vi "TestExec.Run Executable and Rtn.vi"(7 "Vars":variant, 8 "error in":errorcluster, 9 "Timeout(s)":dbl=500.0 caption="Time Out(s)" format="%.2f", 10 "Log Dir":path=path "c:/MTE/Temp", 11 "Input":string[](array[string]) caption="Inputs") -> (0 "Error":errorcluster, 3 "RTN Data":T1 {"MeasData"."Status" items=["LOG", "PASS", "FAIL", "ERROR"]; "Attr"."Status" items=["LOG", "PASS", "FAIL", "ERROR"]; "Num"."Status" items=["LOG", "PASS", "FAIL", "ERROR"]})   [LabVIEW 2024]
uses:
  Cmd Exe/CmdExe.Output Error Check Setup.ctl
  Cmd Exe/CmdExe.Setup Params.ctl
  Results/Result.Measurement and Attribute Item Status.ctl
  Results/Result.Attribute.ctl
  Results/Result.Limit Type.ctl
  Results/Result.Numeric.ctl
  Results/Result XML/TestResult.SW Item.ctl
  Reports/Report.Result FileDataObject.ctl
  TestExec.Local Result Data.ctl
  Errors.lvlib
  <vilib>/KATE/Time/Time Utils.lvlib
  Results/Result.Measurement Item.ctl
  <vilib>/KATE/Files/File Utils.lvlib
panel:
  in  "Tab Control":enum32{"Execute", "Results"}(tab)
  out "Active":bool
  out "Sys Exec Commands":string
  out "Sys Exec STDOut":string
  out "Dur(s)":dbl caption="Duration(s)" format="%.3f"
  out "Rslt":u32(colorbox)=13816530 caption="Exe"
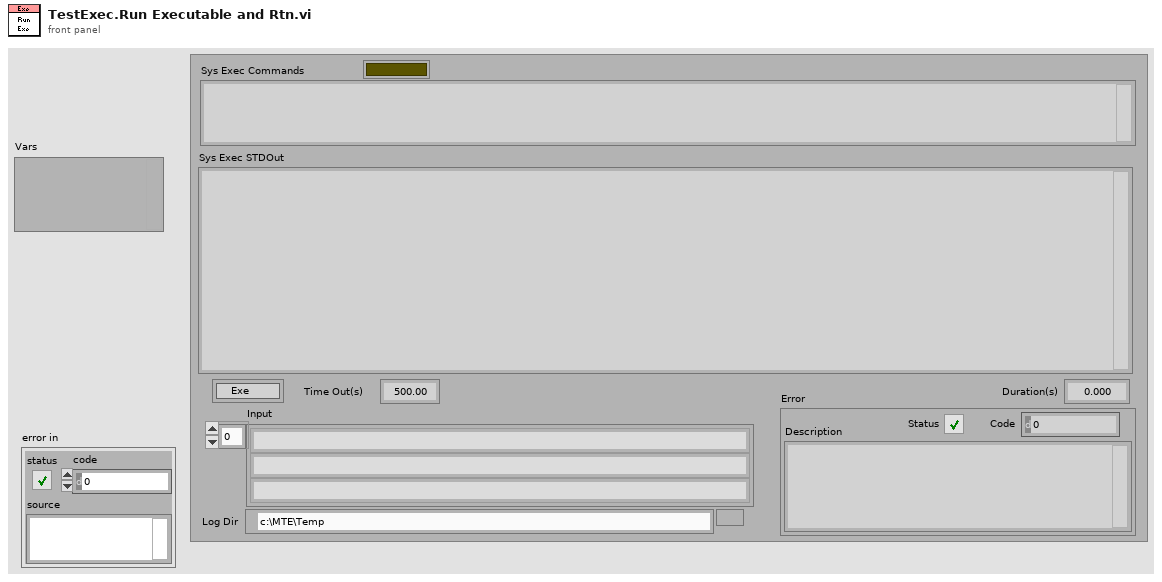
[diagram p1: front panel]
types:
  T1 = typedef "TestExec.Local Result Data.ctl" = cluster{"Attr":T2[], "Num":T4[], "UUT Props":string[][], "Vars":string[][], "SW Items":T6[], "Error":errorcluster, "Step":i32, "FileObjs":T7[], "MeasData":T8[]}
  T2 = typedef "Result.Attribute.ctl" = cluster{"Cnt":i32, "Step":string, "Category":string, "Name":string, "Value":string, "Status":T3, "Code":i32, "Desc":string, "Time":timestamp}
  T3 = typedef "Result.Measurement and Attribute Item Status.ctl" = i32
  T4 = typedef "Result.Numeric.ctl" = cluster{"Cnt":i32, "Step":string, "Category":string, "Name":string, "Value":dbl, "Units":string, "LimType":T5, "LL":dbl, "UL":dbl, "Status":T3, "Code":i32, "Desc":string, "Time":timestamp}
  T5 = typedef "Result.Limit Type.ctl" = enum16{"None", "EQ", "NE", "GT", "LT", "GE", "LE", "GTLT", "GELE", "GELT", "GTLE", "LTGT", "LEGE", "LEGT", "LTGE", "Contains", "NotContains"}
  T6 = typedef "TestResult.SW Item.ctl" = cluster{"Name":string, "PN":string, "Version":string, "Note":string}
  T7 = typedef "Report.Result FileDataObject.ctl" = cluster{"Cnt":i32, "Step":string, "Category":string, "Name":string, "Type":string, "File Name":string, "Time":string, "Path":path}
  T8 = typedef "Result.Measurement Item.ctl" = cluster{"Cnt":i32, "Step":string, "Category":string, "Name":string, "Value":string, "Units":string, "LimType":string, "LL":string, "UL":string, "Status":T3, "Code":i32, "Desc":string, "Time":timestamp}
  T9 = typedef "CmdExe.Setup Params.ctl" = cluster{"Timeout (s)":dbl, "Show Cmd Win":bool, "Error Check":T10, "Log_En":bool, "LogFileName":string, "LogDir":path}
  T10 = typedef "CmdExe.Output Error Check Setup.ctl" = cluster{"StdOut_Ck":bool, "StdOutErrMsgs":string[], "StdErr_Ck":bool, "RtnCode_Ck":bool, "RtnCodePASS":i32}
  T11 = cluster{"Args":string, "Setup":T9, "StdOut":string, "ActionName":string, "Exe":path, "RTN Data":T1, "Prefix":string, "BaseCode":i32, "LogEn":bool, "StdErr":string, "RtnCode":i32}
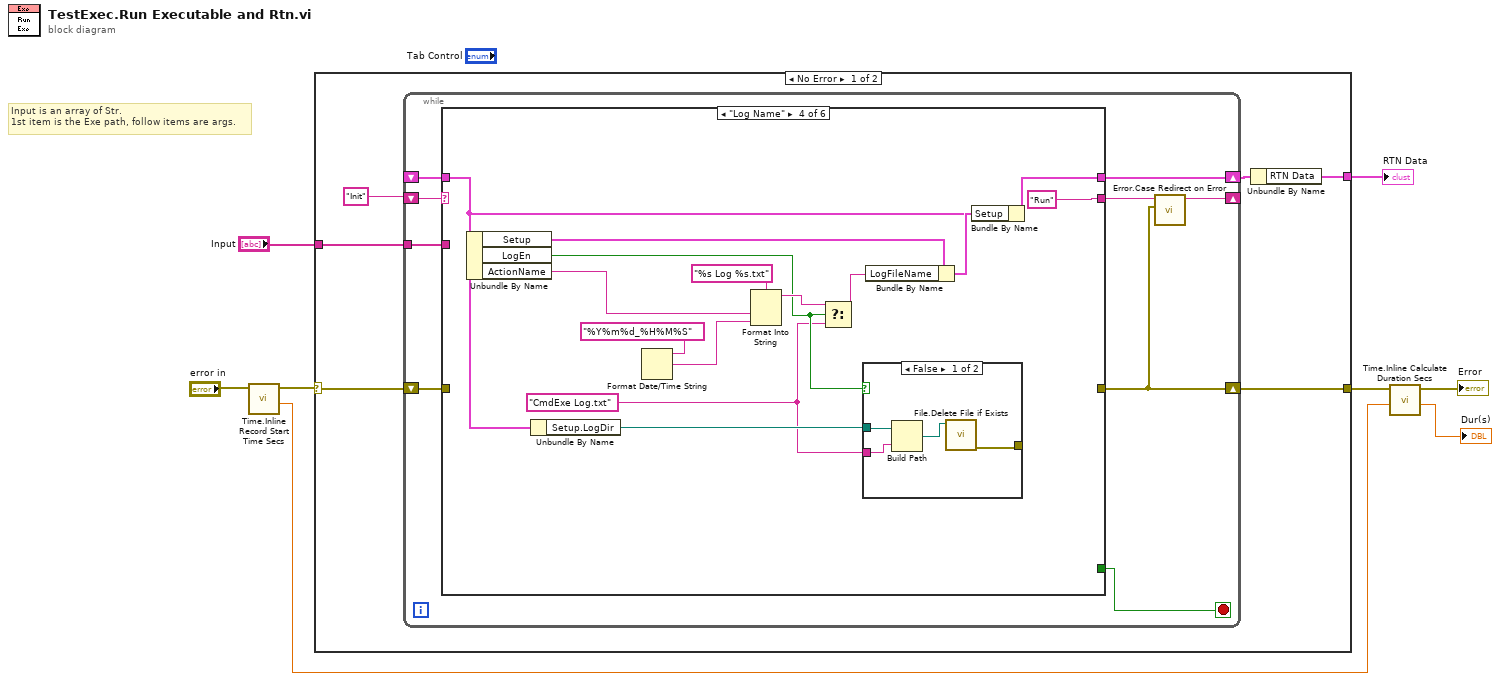
[diagram p0: block diagram]
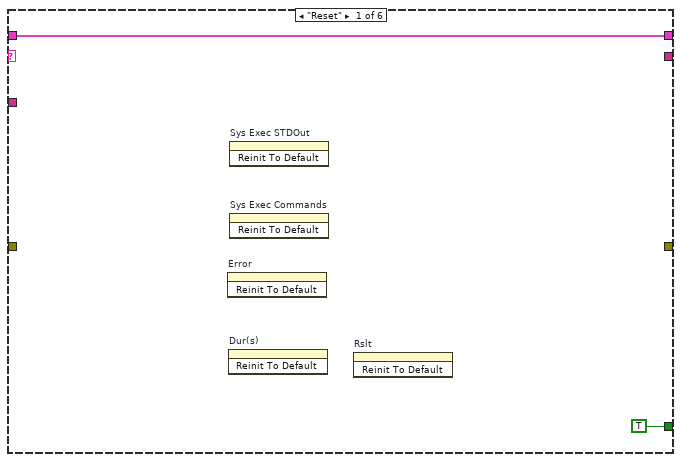
[diagram p2: hidden frame]
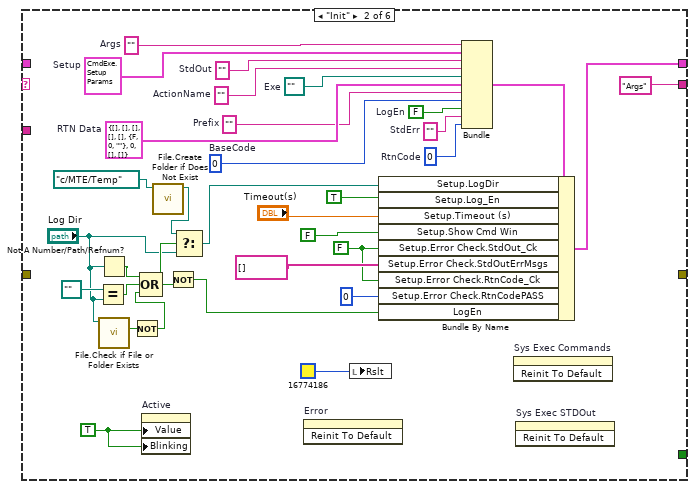
[diagram p3: hidden frame]
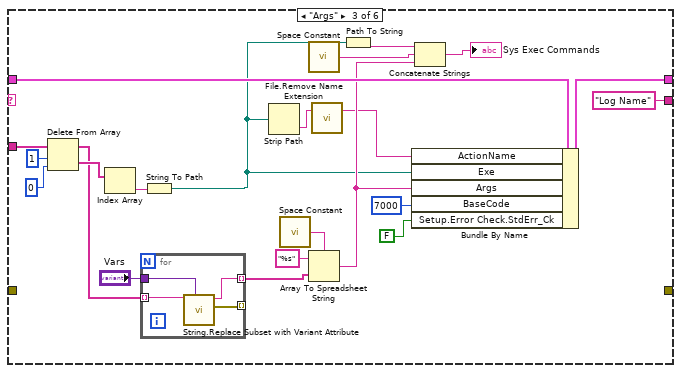
[diagram p4: hidden frame]
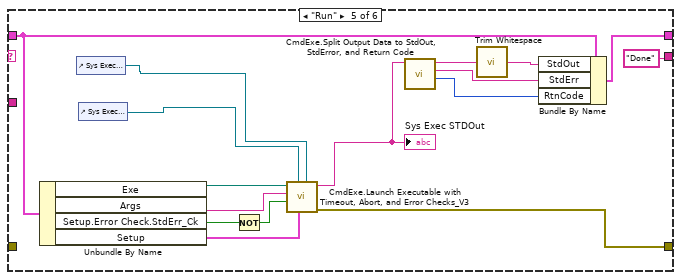
[diagram p6: hidden frame]
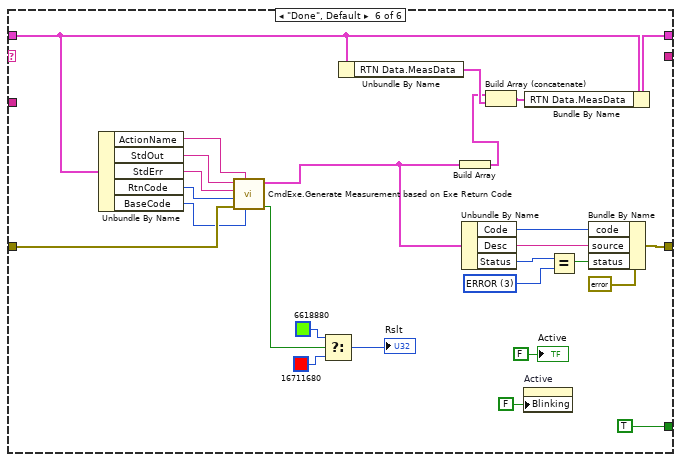
[diagram p7: hidden frame]
diagram:
  # "Input is an array of Str.\n1st item is the Exe path, follow items are args."
  n1 = call <vilib>:"Time.Inline Record Start Time Secs.vi"("Error In Upper"="error in") -> ("Start(s)"=w2:dbl, "Error Out Upper"=w6:errorcluster)  [unwired: 8 in, 1 out]
  n2 = case shown="No Error" w6 {
    selector: w6 -> [w14 w145]
    tunnel: [w13 w145] -> w4
    tunnel: [w11 _] -> w8
    tunnel: "Input" -> [w9 _]
    frame No Error {
      n3 = while {
        shift-right: [w17] -> _
        shift-left: "Init" -> [w23]
        shift-right: [w22] -> w12
        shift-left: _ -> [w21]
        shift-right: [w16] -> w13
        shift-left: w14 -> [w19]
        tunnel: w9 -> [w15]
        stop <- w20 stop-if-true
        n4 = case shown="\"Log Name\"" w23 {
          tunnel: [_ "Args" "Log Name" "Run" "Done" _] -> w18
          tunnel: [w25 w51 w80 w97 w108 w135] -> w22
          tunnel: w21 -> [w25 _ w79 w87 w110 w134]
          tunnel: [TRUE _ _ _ _ TRUE] -> w20
          tunnel: w19 -> [_ _ _ _ _ w129]
          tunnel: [_ _ _ _ w107 w124] -> w16
          tunnel: w15 -> [_ _ w69 _ _ _]
          frame "Reset" {
            n5 = invoke on="Error" class="Clust (strict)" method="Reinit To Default"() -> ()  [unwired: 3 in, 3 out]
            n6 = invoke on="Dur(s)" class="DigNum (strict)" method="Reinit To Default"() -> ()  [unwired: 3 in, 3 out]
            n7 = invoke on="Sys Exec STDOut" class="Str" method="Reinit To Default"() -> ()  [unwired: 3 in, 3 out]
            n8 = invoke on="Sys Exec Commands" class="Str" method="Reinit To Default"() -> ()  [unwired: 3 in, 3 out]
            n9 = invoke on="Rslt" class="ColBox" method="Reinit To Default"() -> ()  [unwired: 3 in, 3 out]
          }
          frame "Init" {
            w28 = 0  # RtnCode
            w29 = ""  # StdErr
            w35 = FALSE  # LogEn
            w42 = 0  # BaseCode
            w43 = ""  # Prefix
            w44 = T1 {"Attr"=[], "Num"=[], "UUT Props"=[], "Vars"=[], "SW Items"=[], "Error"={"status"=FALSE, "code"=0, "source"=""}, "Step"=0, "FileObjs"=[], "MeasData"=[]}  # RTN Data
            w45 = path ""  # Exe
            w46 = ""  # ActionName
            w48 = ""  # StdOut
            w26 = FALSE
            w56 = TRUE ("Value")
            w55 = T9 {"Timeout (s)"=60.0, "Show Cmd Win"=FALSE, "Error Check"={"StdOut_Ck"=FALSE, "StdOutErrMsgs"=["Error", "Unable to find device "], "StdErr_Ck"=FALSE, "RtnCode_Ck"=FALSE, "RtnCodePASS"=0}, "Log_En"=FALSE, "LogFileName"="", "LogDir"=path ""}  # Setup
            w58 = ""  # Args
            n10 = Equal?(x=path "", y="Log Dir") -> (x = y?=w39:bool)
            n11 = Not A Number/Path/Refnum?(number/path/refnum="Log Dir") -> (NaN/Path/Refnum?=w40:bool)
            n12 = call <vilib>:"File.Check if File or Folder Exists.vi"("Path"="Log Dir") -> ("Exists"=w30:bool)  [unwired: 6 in, 4 out]
            n13 = Not(x=w30) -> (.not. x?=w31:bool)
            n14 = Compound Arithmetic op=OR(w40, w39, w31) -> (w34:bool)
            n15 = property on="Active" class="Bool (strict)"("Value"=w56, "Blinking"=w56) -> ()  [unwired: 2 in, 2 out]
            n16 = call <vilib>:"File.Create Folder if Does Not Exist.vi"("Path"=path "c:/MTE/Temp") -> ("Dup Path"=w37:path)  [unwired: 8 in, 2 out]
            n17 = Not(x=w34) -> (.not. x?=w33:bool)
            n18 = Select(t=w37, s=w34, f="Log Dir") -> (s? t:f=w36:path)
            n19 = invoke on="Error" class="Clust (strict)" method="Reinit To Default"() -> ()  [unwired: 3 in, 3 out]
            n20 = local write "Rslt"(u32 16774186) -> ()
            n21 = Bundle("Args"=w58, "Setup"=w55, "StdOut"=w48, "ActionName"=w46, "Exe"=w45, "RTN Data"=w44, "Prefix"=w43, "BaseCode"=w42, "LogEn"=w35, "StdErr"=w29, "RtnCode"=w28) -> (w52:T11)  [unwired: 1 in]
            n22 = Bundle By Name(cluster=w52, "Setup.LogDir"=w36, "Setup.Log_En"=TRUE, "Setup.Timeout (s)"="Timeout(s)", "Setup.Show Cmd Win"=FALSE, "Setup.Error Check.StdOut_Ck"=w26, "Setup.Error Check.StdOutErrMsgs"=string[] [], "Setup.Error Check.RtnCode_Ck"=w26, "Setup.Error Check.RtnCodePASS"=0 ("Error Check.RtnCodePASS"), "LogEn"=w33) -> (w51:T11)
            n23 = invoke on="Sys Exec Commands" class="Str" method="Reinit To Default"() -> ()  [unwired: 3 in, 3 out]
            n24 = invoke on="Sys Exec STDOut" class="Str" method="Reinit To Default"() -> ()  [unwired: 3 in, 3 out]
          }
          frame "Args" {
            n25 = Delete From Array(array=w69, length=1, index=0) -> (deleted portion=w66:string[], array with subset deleted=w63:string[])
            n26 = Index Array(array=w66) -> (element=w65:string)  [unwired: 1 in]
            n27 = for {
              tunnel: "Vars" -> [w84]
              tunnel: w63 -> [w83] mode=indexing
              tunnel: [w82] -> _ mode=indexing
              tunnel: [w81] -> w62 mode=indexing
              n28 = call "String.Replace Subset with Variant Attribute.vi"("Vars"=w84, "Data In"=w83) -> ("error out"=w82:errorcluster, "Data Out"=w81:string)  [unwired: 8 in]
            }
            n29 = String To Path(string=w65) -> (path=w61:path)
            n30 = Strip Path(path=w61) -> (name=w60:string)  [unwired: 1 out]
            n31 = call <vilib>:"Space Constant.vi"() -> ("String"=w76:string)
            n32 = call <vilib>:"Space Constant.vi"() -> ("String"=w72:string)
            n33 = Array To Spreadsheet String(delimiter (Tab)=w76, array=w62, 3:"%s" ("format string")) -> (spreadsheet string=w73:string)
            n34 = call <vilib>:"File.Remove Name Extension.vi"("File Name"=w60) -> ("Name Less Ext"=w59:string)  [unwired: 1 in, 1 out]
            n35 = Path To String(path=w61) -> (string=w74:string)
            n36 = Bundle By Name(cluster=w79, "ActionName"=w59, "Exe"=w61, "Args"=w73, "BaseCode"=7000 ("Code"), "Setup.Error Check.StdErr_Ck"=FALSE) -> (w80:T11)
            n37 = Concatenate Strings(w74, w72, w73) -> (→"Sys Exec Commands":string)
          }
          frame "Log Name" {
            w85 = "CmdExe Log.txt"
            n38 = Unbundle By Name(w87) -> ("Setup"=w95:T9, "LogEn"=w88:bool, "ActionName"=w91:string)
            n39 = Unbundle By Name(w87) -> ("Setup.LogDir"=w86:path)
            n40 = Format Date/Time String(time format string (%c)="%Y%m%d_%H%M%S") -> (date/time string=w92:string)  [unwired: 2 in]
            n41 = Format Into String(format string="%s Log %s.txt", w91, w92) -> (resulting string=w90:string)  [unwired: 2 in, 1 out]
            n42 = Select(t=w90, s=w88, f=w85) -> (s? t:f=w89:string)
            n43 = case shown="False" w88 {
              tunnel: w86 -> [w102 _]
              tunnel: w85 -> [w101 _]
              tunnel: [w99 _] -> _
              frame False {
                n44 = Build Path(base path=w102, name or relative path=w101) -> (appended path=w100:path)
                n45 = call "File.Delete File if Exists.vi"("Path"=w100) -> ("error out"=w99:errorcluster)  [unwired: 9 in, 1 out]
              }
              frame True {
              }
            }
            n46 = Bundle By Name(cluster=w95, "LogFileName"=w89) -> (w96:T9)
            n47 = Bundle By Name(cluster=w87, "Setup"=w96) -> (w97:T11)
          }
          frame "Run" {
            n48 = Unbundle By Name(w110) -> ("Exe"=w109:path, "Args"=w118:string, "Setup.Error Check.StdErr_Ck"=w106:bool, "Setup"=w117:T9)
            n49 = control-ref of="Sys Exec Commands"() -> (w116:refnum<vi>)
            n50 = control-ref of="Sys Exec STDOut"() -> (w115:refnum<vi>)
            n51 = Not(x=w106) -> (.not. x?=w105:bool)
            n52 = call "CmdExe.Launch Executable with Timeout, Abort, and Error Checks_V3.vi"("Cmd IN Ref"=w116, "Setup"=w117, "Output Ref"=w115, "Ignore StdErr"=w105, "Args"=w118, "Executable"=w109) -> ("error out"=w107:errorcluster, "Data Out"=w112:string)  [unwired: 2 in, 2 out]
            "Sys Exec STDOut" <- w112
            n53 = call "CmdExe.Split Output Data to StdOut, StdError, and Return Code.vi"("Output Data"=w112) -> ("Return Code"=w103:i32, "StdError"=w104:string, "StdOut"=w113:string)  [unwired: 7 in, 1 out]
            n54 = call <vilib>:"Trim Whitespace.vi"("string"=w113) -> ("trimmed string"=w111:string)  [unwired: 1 in]
            n55 = Bundle By Name(cluster=w110, "StdOut"=w111, "StdErr"=w104, "RtnCode"=w103) -> (w108:T11)
          }
          frame "Done", Default {
            w120 = T3 3 items=["LOG", "PASS", "FAIL", "ERROR"] ("Status")
            n56 = Unbundle By Name(w134) -> ("ActionName"=w133:string, "StdOut"=w132:string, "StdErr"=w131:string, "RtnCode"=w130:i32, "BaseCode"=w127:i32)
            n57 = call "CmdExe.Generate Measurement based on Exe Return Code.vi"("BaseCode"=w127, "Name"=w133, "Error"=w129, "RtnCode"=w130, "StdErr"=w131, "StdOut"=w132) -> ("Success"=w128:bool, "Meas"=w126:T8)  [unwired: 4 in]
            n58 = Select(t=u32 6618880, s=w128, f=u32 16711680) -> (s? t:f=→"Rslt":u32)
            n59 = Unbundle By Name(w134) -> ("RTN Data.MeasData"=w138:T8[])
            n60 = Build Array(w126) -> (w137:T8[])
            n61 = Unbundle By Name(w126) -> ("Code"=w122:i32, "Desc"=w123:string, "Status"=w121:T3)
            n62 = Build Array (concatenate)(w137, w138) -> (w139:T8[])
            n63 = property on="Active" class="Bool (strict)"("Blinking"=FALSE ("Value")) -> ()  [unwired: 2 in, 2 out]
            n64 = Bundle By Name(cluster=w134, "RTN Data.MeasData"=w139) -> (w135:T11)
            n65 = Equal?(x=w121, y=w120) -> (x = y?=w119:bool)
            n66 = Bundle By Name(cluster=errorcluster {"status"=FALSE, "code"=0, "source"=""} ("error constant"), "code"=w122, "source"=w123, "status"=w119) -> (w124:errorcluster)
            "Active" <- FALSE ("Active")
          }
        }
        n67 = call "Error.Case Redirect on Error.vi"("error in"=w16, "Next Case"=w18) -> ("Next Case Out"=w17:string)  [unwired: 9 in]
      }
      n68 = Unbundle By Name(w12) -> ("RTN Data"=w11:T1)
    }
    frame Error {
    }
  }
  "RTN Data" <- w8
  n69 = call <vilib>:"Time.Inline Calculate Duration Secs.vi"("Start(Sec)"=w2, "Error In Top"=w4) -> ("Duration(s)"=→"Dur(s)":dbl, "Error Out Top"=→"Error":errorcluster)  [unwired: 7 in, 1 out]
